vi "FT_Status to Error.vi"(8 "error in (no error)":errorcluster, 11 "Numeric":i32) -> (0 "error out":errorcluster)   [LabVIEW 2019]
uses:
  <userlib>/LevyLab/Relay Box/D2XX_Functions/D2XX_Functions.lvlib
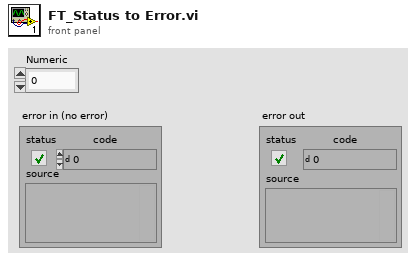
[diagram p1: front panel]
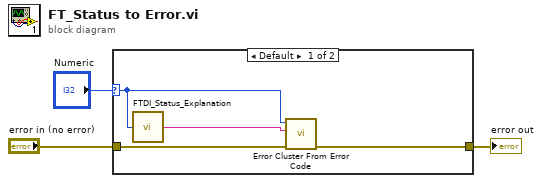
[diagram p0: block diagram]
diagram:
  n1 = case shown="Default" "Numeric" {
    selector: "Numeric" -> [w4 _]
    tunnel: "error in (no error)" -> [w6 w8]
    tunnel: [w5 w8] -> w2
    frame Default {
      n2 = call <userlib>:"FTDI_Status_Explanation.vi"("FT_Status"=w4) -> ("Status String"=w7:string)
      n3 = call <vilib>:"Error Cluster From Error Code.vi"("error in (no error)"=w6, "error message (\"\")"=w7, "error code (0)"=w4) -> ("error out"=w5:errorcluster)  [unwired: 6 in]
    }
    frame 1 {
    }
  }
  "error out" <- w2
